vi "Set CFG wrapper.vi"(7 "UIM_MCFG_INFO_OBJ In":T1, 8 "error in (no error)":errorcluster caption="错误输入（无错误）", 9 "UIM_ICFG_INFO_OBJ In":T2, 10 "dwCanNodeId":u32, 11 "dwDevIndex":u32) -> (0 "error out":errorcluster caption="错误输出", 1 "UIM_ICFG_INFO_OBJ Out":T2, 3 "function return":u32, 5 "UIM_MCFG_INFO_OBJ Out":T1)   [LabVIEW 2016, in "UISimCanFunc_wrapper.lvlib"]
doc: "_declspec (dllexport) DWORD SetCFG_wrapper(DWORD dwDevIndex, DWORD dwCanNodeId,\n P_DUMMY_UIM_ICFG_INFO_OBJ pDummyICFGInfoOut, P_DUMMY_UIM_MCFG_INFO_OBJ pDummyMCFGInfo);"
uses:
  <userlib>/UISimCanFunc_wrapper/UISimCanFunc_wrapper.lvlib
  <userlib>/UISimCanFunc_wrapper/ctl/UIM_ICFG_INFO_OBJ.ctl
  <userlib>/UISimCanFunc_wrapper/ctl/UIM_MCFG_INFO_OBJ.ctl
  <userlib>/UISimCanFunc_wrapper/UISimCanFunc_wrapper.dll
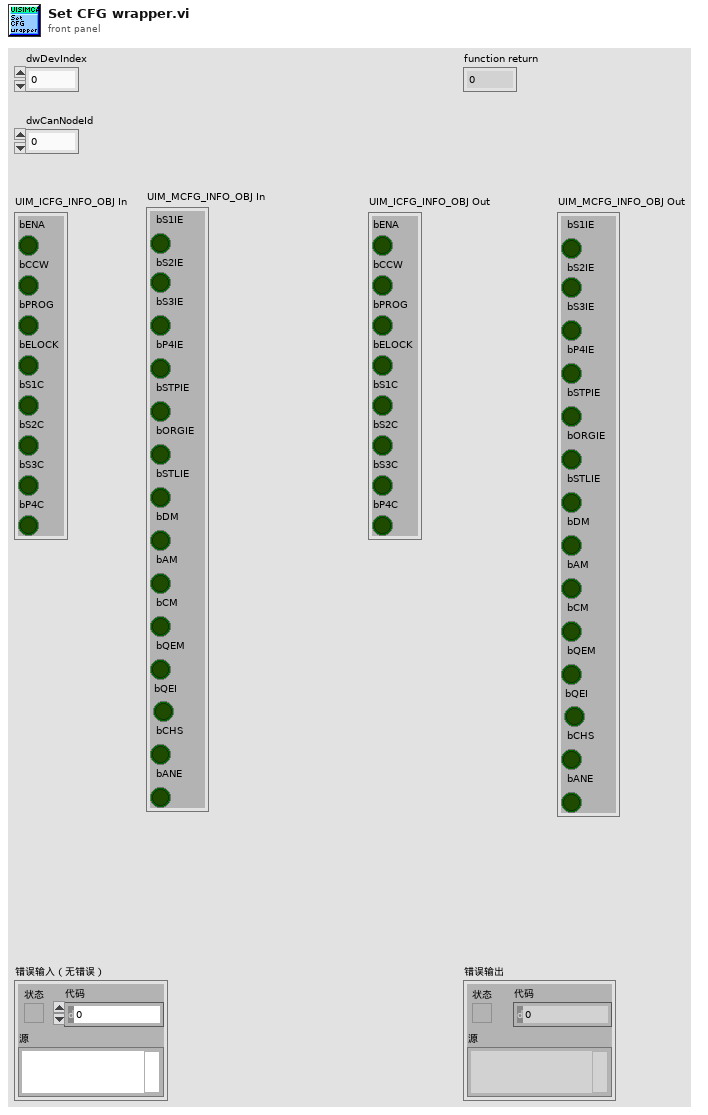
[diagram p1: front panel]
types:
  T1 = typedef "UISimCanFunc_wrapper.lvlib/UIM_MCFG_INFO_OBJ.ctl" = cluster{" bS1IE":bool, " bS2IE":bool, " bS3IE":bool, " bP4IE":bool, " bSTPIE":bool, " bORGIE":bool, " bSTLIE":bool, " bDM":bool, " bAM":bool, " bCM":bool, " bQEM":bool, " bQEI        ":bool, " bCHS":bool, " bANE":bool}
  T2 = typedef "UISimCanFunc_wrapper.lvlib/UIM_ICFG_INFO_OBJ.ctl" = cluster{"bENA":bool, "bCCW":bool, "bPROG":bool, "bELOCK":bool, "bS1C":bool, "bS2C":bool, "bS3C":bool, "bP4C":bool}
  T3 = cluster{"bENA":i32, "bCCW":i32, "bPROG":i32, "bELOCK":i32, "bS1C":i32, "bS2C":i32, "bS3C":i32, "bP4C":i32}
  T4 = cluster{"bS1IE":i32, "bS2IE":i32, "bS3IE":i32, "bP4IE":i32, "bSTPIE":i32, "bORGIE":i32, "bSTLIE":i32, "bDM":i32, "bAM":i32, "bCM":i32, "bQEM":i32, "bQEI":i32, "bCHS":i32, "bANE":i32}
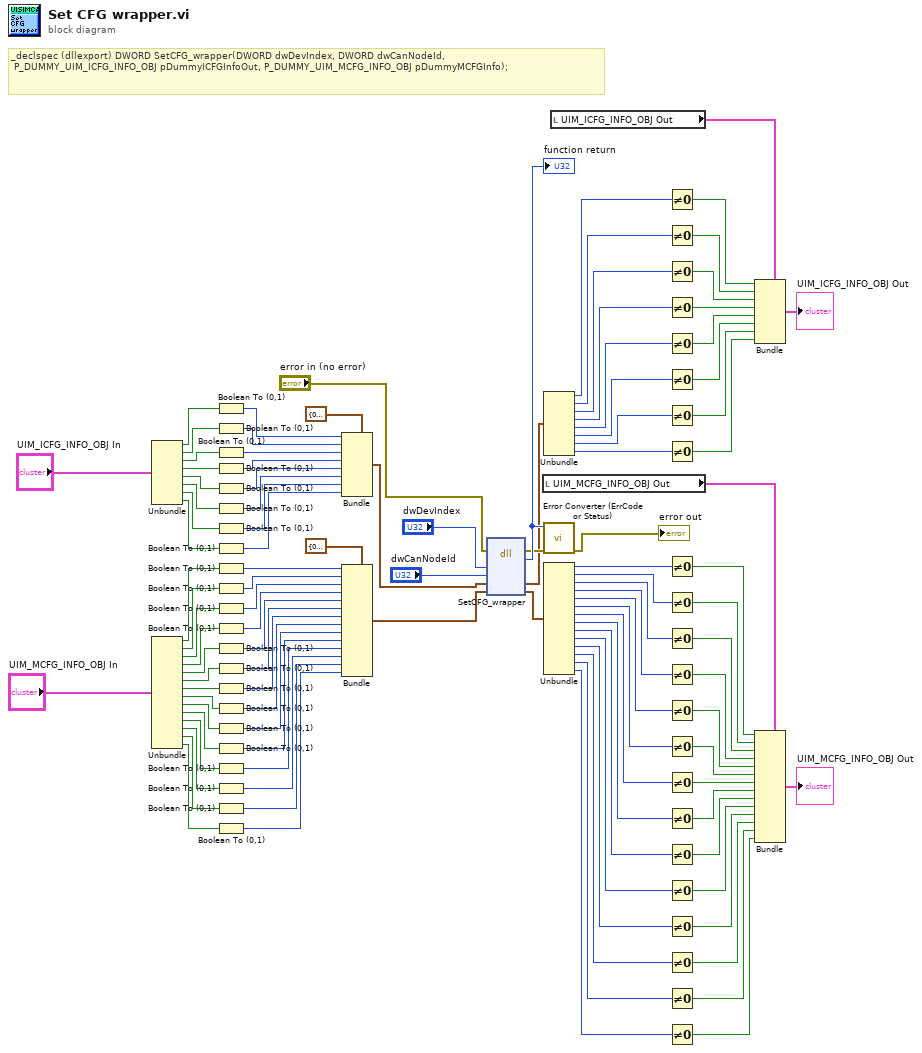
[diagram p0: block diagram]
diagram:
  # "_declspec (dllexport) DWORD SetCFG_wrapper(DWORD dwDevIndex, DWORD dwCanNodeId,\n\tP_DUMMY_UIM_ICFG_INFO_OBJ pDummyICFGInfoOut, P_DUMMY_UIM_MCFG_INFO_OBJ pDummyMCFGInfo);"
  n1 = Unbundle("UIM_ICFG_INFO_OBJ In") -> ("bENA"=w98:bool, "bCCW"=w97:bool, "bPROG"=w96:bool, "bELOCK"=w95:bool, "bS1C"=w16:bool, "bS2C"=w15:bool, "bS3C"=w14:bool, "bP4C"=w13:bool)
  n2 = Unbundle("UIM_MCFG_INFO_OBJ In") -> ("bS1IE"=w87:bool, "bS2IE"=w86:bool, "bS3IE"=w85:bool, "bP4IE"=w84:bool, "bSTPIE"=w83:bool, "bORGIE"=w82:bool, "bSTLIE"=w81:bool, "bDM"=w80:bool, "bAM"=w79:bool, "bCM"=w78:bool, "bQEM"=w77:bool, "bQEI"=w76:bool, "bCHS"=w75:bool, "bANE"=w74:bool)
  n3 = Boolean To (0,1)(Boolean=w98) -> (0, 1=w94:i16)
  n4 = Boolean To (0,1)(Boolean=w97) -> (0, 1=w93:i16)
  n5 = Boolean To (0,1)(Boolean=w96) -> (0, 1=w92:i16)
  n6 = Boolean To (0,1)(Boolean=w95) -> (0, 1=w91:i16)
  n7 = Boolean To (0,1)(Boolean=w16) -> (0, 1=w12:i16)
  n8 = Boolean To (0,1)(Boolean=w15) -> (0, 1=w11:i16)
  n9 = Boolean To (0,1)(Boolean=w14) -> (0, 1=w10:i16)
  n10 = Boolean To (0,1)(Boolean=w13) -> (0, 1=w9:i16)
  n11 = Boolean To (0,1)(Boolean=w87) -> (0, 1=w73:i16)
  n12 = Boolean To (0,1)(Boolean=w86) -> (0, 1=w72:i16)
  n13 = Boolean To (0,1)(Boolean=w85) -> (0, 1=w71:i16)
  n14 = Boolean To (0,1)(Boolean=w84) -> (0, 1=w70:i16)
  n15 = Boolean To (0,1)(Boolean=w83) -> (0, 1=w69:i16)
  n16 = Boolean To (0,1)(Boolean=w82) -> (0, 1=w68:i16)
  n17 = Boolean To (0,1)(Boolean=w81) -> (0, 1=w67:i16)
  n18 = Boolean To (0,1)(Boolean=w80) -> (0, 1=w66:i16)
  n19 = Boolean To (0,1)(Boolean=w79) -> (0, 1=w65:i16)
  n20 = Boolean To (0,1)(Boolean=w78) -> (0, 1=w64:i16)
  n21 = Boolean To (0,1)(Boolean=w77) -> (0, 1=w63:i16)
  n22 = Boolean To (0,1)(Boolean=w76) -> (0, 1=w62:i16)
  n23 = Boolean To (0,1)(Boolean=w75) -> (0, 1=w61:i16)
  n24 = Boolean To (0,1)(Boolean=w74) -> (0, 1=w60:i16)
  n25 = Bundle(cluster=T3 {"bENA"=0, "bCCW"=0, "bPROG"=0, "bELOCK"=0, "bS1C"=0, "bS2C"=0, "bS3C"=0, "bP4C"=0} ("pDummyICFGInfoOut"), "bENA"=w94, "bCCW"=w93, "bPROG"=w92, "bELOCK"=w91, "bS1C"=w12, "bS2C"=w11, "bS3C"=w10, "bP4C"=w9) -> (w99:T3)
  n26 = Bundle(cluster=T4 {"bS1IE"=0, "bS2IE"=0, "bS3IE"=0, "bP4IE"=0, "bSTPIE"=0, "bORGIE"=0, "bSTLIE"=0, "bDM"=0, "bAM"=0, "bCM"=0, "bQEM"=0, "bQEI"=0, "bCHS"=0, "bANE"=0} ("pDummyMCFGInfo"), "bS1IE"=w73, "bS2IE"=w72, "bS3IE"=w71, "bP4IE"=w70, "bSTPIE"=w69, "bORGIE"=w68, "bSTLIE"=w67, "bDM"=w66, "bAM"=w65, "bCM"=w64, "bQEM"=w63, "bQEI"=w62, "bCHS"=w61, "bANE"=w60) -> (w88:T4)
  n27 = dll-call lib="C:/Program Files (x86)/National Instruments/LabVIEW 2016/user.lib/UISimCanFunc_wrapper/UISimCanFunc_wrapper.*" fn="SetCFG_wrapper"(error in="error in (no error)", "dwDevIndex"="dwDevIndex", "dwCanNodeId"="dwCanNodeId", "pDummyICFGInfoOut"=w99, "pDummyMCFGInfo"=w88) -> (error out=w102:errorcluster, w106:u32, "pDummyICFGInfoOut"=w59:T3, "pDummyMCFGInfo"=w58:T4)  [unwired: 4 in, 1 out]
  "function return" <- w106
  n28 = local read "UIM_MCFG_INFO_OBJ Out"() -> (w55:T1)
  n29 = Unbundle(w59) -> ("bENA"=w53:i32, "bCCW"=w52:i32, "bPROG"=w51:i32, "bELOCK"=w50:i32, "bS1C"=w8:i32, "bS2C"=w7:i32, "bS3C"=w6:i32, "bP4C"=w5:i32)
  n30 = call <userlib>:"Error Converter (ErrCode or Status).vi"("error in (no error)"=w102, "error code"=w106) -> ("error out"=→"error out":errorcluster)  [unwired: 9 in]
  n31 = Unbundle(w58) -> ("bS1IE"=w45:i32, "bS2IE"=w44:i32, "bS3IE"=w43:i32, "bP4IE"=w42:i32, "bSTPIE"=w41:i32, "bORGIE"=w40:i32, "bSTLIE"=w39:i32, "bDM"=w38:i32, "bAM"=w37:i32, "bCM"=w36:i32, "bQEM"=w35:i32, "bQEI"=w34:i32, "bCHS"=w33:i32, "bANE"=w32:i32)
  n32 = local read "UIM_ICFG_INFO_OBJ Out"() -> (w57:T2)
  n33 = Not Equal To 0?(x=w53) -> (x != 0?=w49:bool)
  n34 = Not Equal To 0?(x=w52) -> (x != 0?=w48:bool)
  n35 = Not Equal To 0?(x=w51) -> (x != 0?=w47:bool)
  n36 = Not Equal To 0?(x=w50) -> (x != 0?=w46:bool)
  n37 = Not Equal To 0?(x=w8) -> (x != 0?=w4:bool)
  n38 = Not Equal To 0?(x=w7) -> (x != 0?=w3:bool)
  n39 = Not Equal To 0?(x=w6) -> (x != 0?=w2:bool)
  n40 = Not Equal To 0?(x=w5) -> (x != 0?=w1:bool)
  n41 = Not Equal To 0?(x=w45) -> (x != 0?=w31:bool)
  n42 = Not Equal To 0?(x=w44) -> (x != 0?=w30:bool)
  n43 = Not Equal To 0?(x=w43) -> (x != 0?=w29:bool)
  n44 = Not Equal To 0?(x=w42) -> (x != 0?=w28:bool)
  n45 = Not Equal To 0?(x=w41) -> (x != 0?=w27:bool)
  n46 = Not Equal To 0?(x=w40) -> (x != 0?=w26:bool)
  n47 = Not Equal To 0?(x=w39) -> (x != 0?=w25:bool)
  n48 = Not Equal To 0?(x=w38) -> (x != 0?=w24:bool)
  n49 = Not Equal To 0?(x=w37) -> (x != 0?=w23:bool)
  n50 = Not Equal To 0?(x=w36) -> (x != 0?=w22:bool)
  n51 = Not Equal To 0?(x=w35) -> (x != 0?=w21:bool)
  n52 = Not Equal To 0?(x=w34) -> (x != 0?=w20:bool)
  n53 = Not Equal To 0?(x=w33) -> (x != 0?=w19:bool)
  n54 = Not Equal To 0?(x=w32) -> (x != 0?=w18:bool)
  n55 = Bundle(cluster=w57, "bENA"=w49, "bCCW"=w48, "bPROG"=w47, "bELOCK"=w46, "bS1C"=w4, "bS2C"=w3, "bS3C"=w2, "bP4C"=w1) -> (→"UIM_ICFG_INFO_OBJ Out":T2)
  n56 = Bundle(cluster=w55, "bS1IE"=w31, "bS2IE"=w30, "bS3IE"=w29, "bP4IE"=w28, "bSTPIE"=w27, "bORGIE"=w26, "bSTLIE"=w25, "bDM"=w24, "bAM"=w23, "bCM"=w22, "bQEM"=w21, "bQEI"=w20, "bCHS"=w19, "bANE"=w18) -> (→"UIM_MCFG_INFO_OBJ Out":T1)
